vi "Get Instrument Alias.vi"(8 "error in (no error)":errorcluster, 11 "SDG1032X in":refnum<class "SDG1032X.lvclass">) -> (0 "error out":errorcluster, 2 "Instrument Alias":string, 3 "SDG1032X out":refnum<class "SDG1032X.lvclass">)   [LabVIEW 2023, in "HAF.lvlib" / "SDG1032X.lvclass"]
doc: "Returns the alias name of the Instrument for this Driver that can be used to initiate a session. Must be implemented by Subclasses because there is no Visa Session available to obtain it from when it is needed.\n\nIt's not ideal: need to think of a better way of dealing with attached resources than hard-coded aliases which must match what was entered in NI-MAX."
uses:
  SDG1032X.lvclass
  SDG1032X.lvclass/SDG1032X.ctl
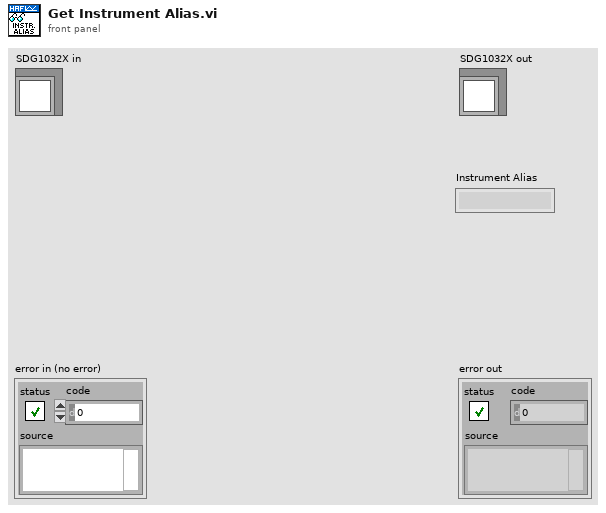
[diagram p1: front panel]
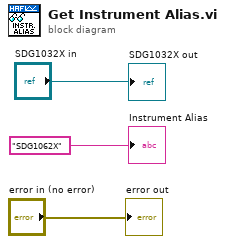
[diagram p0: block diagram]
diagram:
  "error out" <- "error in (no error)"
  "SDG1032X out" <- "SDG1032X in"
  "Instrument Alias" <- "SDG1062X" ("Instrument Alias")
